vi "GOOP_LVClass_CreateNewWizard_GetCreateNewWeight.vi"(11 "Wizard":u64) -> (3 "Weight":i32)   [LabVIEW 2014]
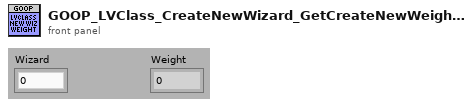
[diagram p1: front panel]
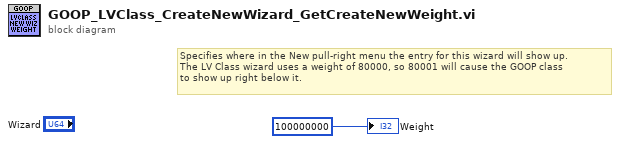
[diagram p0: block diagram]
diagram:
  # "Specifies where in the New pull-right menu the entry for this wizard will show up. \nThe LV Class wizard uses a weight of 80000, so 80001 will cause the GOOP class\nto show up right below it."
  "Weight" <- 100000000 ("Weight")
